vi "Poll.ConvertChannelsToString.vi"(8 "error in (no error)":errorcluster, 11 "MonitoredChannelSettings":T1) -> (0 "error out":errorcluster, 3 "Array":string[](array[string]))   [LabVIEW 2019, in "Diagnostics Addon System Explorer.lvlib"]
uses:
  Diagnostics Addon System Explorer.lvlib
  Types/Poll.LinkedNode.ctl
  <vilib>/NI VeriStand/Custom Device API/Custom Device API.lvlib
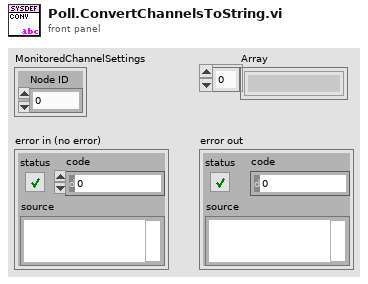
[diagram p1: front panel]
types:
  T1 = typedef "Diagnostics Addon System Explorer.lvlib/Poll.LinkedNode.ctl" = cluster{"Node ID":u64}
  T2 = typedef "Custom Device API.lvlib/Custom Device Item Info.ctl" = cluster{"Name":string, "Is Channel":bool, "GUID":string, "Is Waveform":bool}
  T3 = typedef "Custom Device API.lvlib/Custom Device Item Ref.ctl" = u64
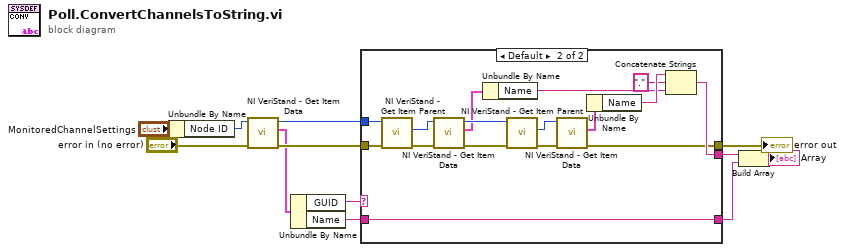
[diagram p0: block diagram]
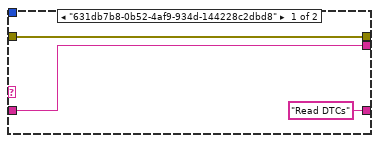
[diagram p2: hidden frame]
diagram:
  n1 = Unbundle By Name("MonitoredChannelSettings") -> ("Node ID"=w5:u64)
  n2 = call <vilib>:"NI VeriStand - Get Item Data.vi"("error in (no error)"="error in (no error)", "Item Ref in"=w5) -> ("error out"=w6:errorcluster, "Item Info"=w3:T2, "Item Ref out"=w9:T3)  [unwired: 7 out]
  n3 = Unbundle By Name(w3) -> ("GUID"=w10:string, "Name"=w12:string)
  n4 = case shown="Default" w10 {
    tunnel: w6 -> [w15 w31]
    tunnel: [w14 w19] -> w7
    tunnel: [w15 w18] -> w8
    tunnel: w9 -> [_ w17]
    tunnel: ["Read DTCs" ("Name") w16] -> w11
    tunnel: w12 -> [w14 w16]
    frame "631db7b8-0b52-4af9-934d-144228c2dbd8" {
    }
    frame Default {
      n5 = call <vilib>:"NI VeriStand - Get Item Parent.vi"("error in (no error)"=w31, "Item Ref in"=w17) -> ("error out"=w30:errorcluster, "Parent Ref"=w29:T3)  [unwired: 6 in, 2 out]
      n6 = call <vilib>:"NI VeriStand - Get Item Data.vi"("error in (no error)"=w30, "Item Ref in"=w29) -> ("error out"=w28:errorcluster, "Item Info"=w24:T2, "Item Ref out"=w27:T3)  [unwired: 7 out]
      n7 = Unbundle By Name(w24) -> ("Name"=w20:string)
      n8 = call <vilib>:"NI VeriStand - Get Item Parent.vi"("error in (no error)"=w28, "Item Ref in"=w27) -> ("error out"=w25:errorcluster, "Parent Ref"=w26:T3)  [unwired: 6 in, 2 out]
      n9 = call <vilib>:"NI VeriStand - Get Item Data.vi"("error in (no error)"=w25, "Item Ref in"=w26) -> ("error out"=w18:errorcluster, "Item Info"=w23:T2)  [unwired: 8 out]
      n10 = Unbundle By Name(w23) -> ("Name"=w22:string)
      n11 = Concatenate Strings(w22, "." ("string"), w20) -> (w19:string)
    }
  }
  "error out" <- w8
  n12 = Build Array(w7, w11) -> (→"Array":string[])
